vi "XML getApiRequest.vi"(11 "Formatted XML":string) -> (3 "PIM API Request":T1={"#attributes"={"xmlns"="http://www.summitekinstruments.com", "xmlns:xsi"="http://www.w3.org/2001/XMLSchema-instance", "xsi:schemaLocation"="http://www.summitekinstruments.com PIMXMLSchema.xsd"}, "Commands"={"#attributes"={"Token"="", "Legacy"=FALSE}, "Command"=[]}})   [LabVIEW 2011]
uses:
  Controls/PIM.API.REQUEST.ctl
  Controls/PIM.API.Command.Collection.ctl
  Controls/PIM.API.Command.Unique.ctl
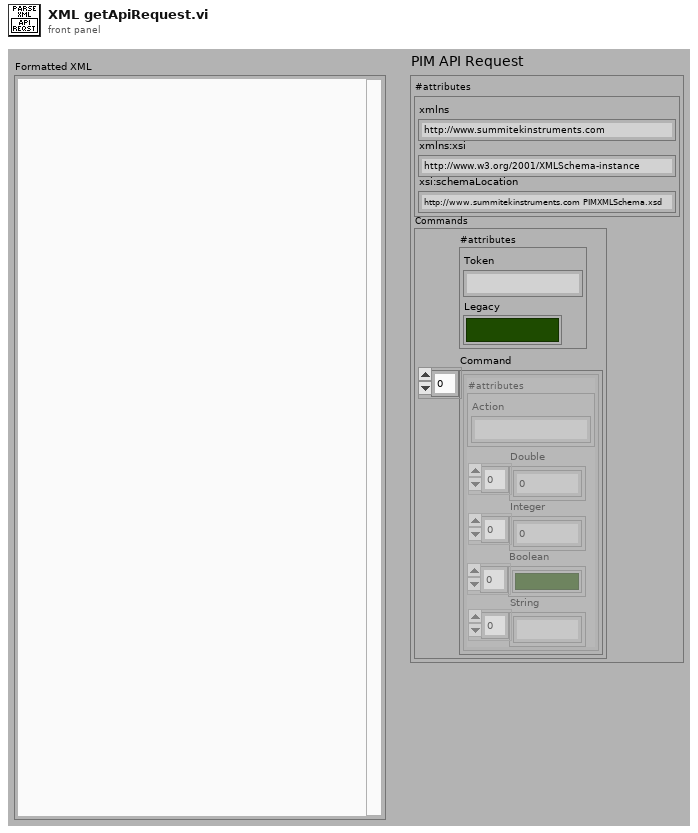
[diagram p1: front panel]
types:
  T1 = typedef "PIM.API.REQUEST.ctl" = cluster{"#attributes":cluster{"xmlns":string, "xmlns:xsi":string, "xsi:schemaLocation":string}, "Commands":T2}
  T2 = typedef "PIM.API.Command.Collection.ctl" = cluster{"#attributes":cluster{"Token":string, "Legacy":bool}, "Command":T3[]}
  T3 = typedef "PIM.API.Command.Unique.ctl" = cluster{"#attributes":cluster{"Action":string}, "Double":dbl[], "Integer":i32[], "Boolean":bool[], "String":string[]}
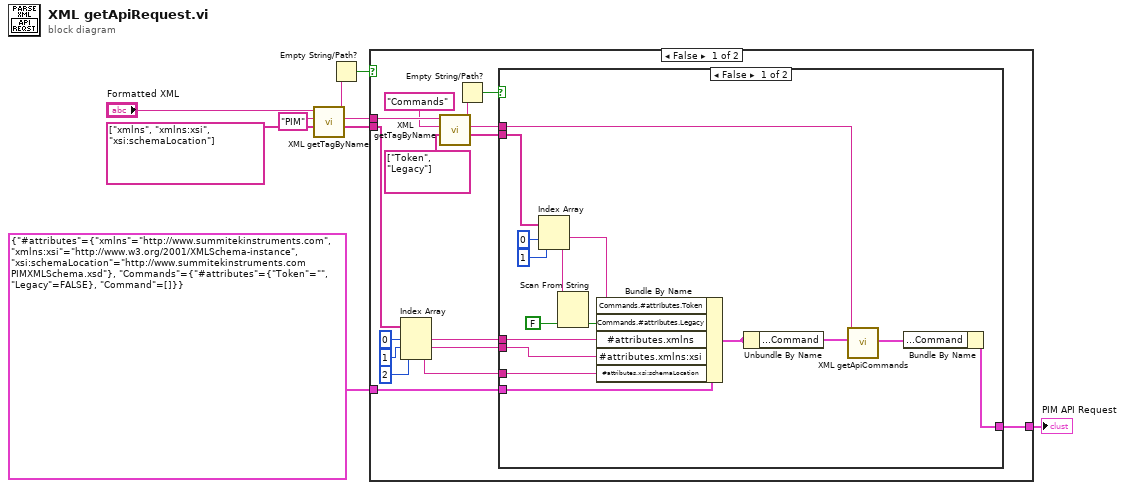
[diagram p0: block diagram]
diagram:
  n1 = call "XML getTagByName.vi"("Get Attributes"=string[] ["xmlns", "xmlns:xsi", "xsi:schemaLocation"], "Tag Name"="PIM", "XML String"="Formatted XML") -> ("Attribute Values"=w3:string[], "Tag Contents"=w2:string, "Matching Tag"=w1:string)  [unwired: 4 in, 2 out]
  n2 = Empty String/Path?(string/path=w1) -> (empty?=w9:bool)
  n3 = case shown="False" w9 {
    tunnel: T1 {"#attributes"={"xmlns"="http://www.summitekinstruments.com", "xmlns:xsi"="http://www.w3.org/2001/XMLSchema-instance", "xsi:schemaLocation"="http://www.summitekinstruments.com PIMXMLSchema.xsd"}, "Commands"={"#attributes"={"Token"="", "Legacy"=FALSE}, "Command"=[]}} ("PIM API Request") -> [w17 w43]
    tunnel: [w10 w43] -> w7
    tunnel: w2 -> [w25 _]
    tunnel: w3 -> [w21 _]
    frame False {
      n4 = Index Array(array=w21, index #1=0 ("index"), index #2=1 ("index"), index #3=2 ("index")) -> (element #1=w20:string, element #2=w19:string, element #3=w18:string)
      n5 = call "XML getTagByName.vi"("Get Attributes"=string[] ["Token", "Legacy"], "Tag Name"="Commands", "XML String"=w25) -> ("Attribute Values"=w13:string[], "Tag Contents"=w23:string, "Matching Tag"=w12:string)  [unwired: 4 in, 2 out]
      n6 = Empty String/Path?(string/path=w12) -> (empty?=w11:bool)
      n7 = case shown="False" w11 {
        tunnel: w23 -> [w26 _]
        tunnel: w20 -> [w41 _]
        tunnel: w19 -> [w40 _]
        tunnel: w18 -> [w39 _]
        tunnel: w17 -> [w38 w42]
        tunnel: w13 -> [w30 _]
        tunnel: [w27 w42] -> w10
        frame False {
          n8 = Index Array(array=w30, index #1=0 ("index"), index #2=1 ("index")) -> (element #1=w36:string, element #2=w33:string)
          n9 = Scan From String(input string=w33, default 1=FALSE ("Legacy")) -> (output 1=w32:bool)  [unwired: 3 in, 3 out]
          n10 = Bundle By Name(cluster=w38, "Commands.#attributes.Token"=w36, "Commands.#attributes.Legacy"=w32, "#attributes.xmlns"=w41, "#attributes.xmlns:xsi"=w40, "#attributes.xsi:schemaLocation"=w39) -> (w29:T1)
          n11 = Unbundle By Name(w29) -> ("Commands.Command"=w31:T3[])
          n12 = call "XML getApiCommands.vi"("Commands In"=w31, "Commands XML"=w26) -> ("Commands Out"=w28:T3[])  [unwired: 9 in]
          n13 = Bundle By Name(cluster=w29, "Commands.Command"=w28) -> (w27:T1)
        }
        frame True {
        }
      }
    }
    frame True {
      # "Tag Not Found"
    }
  }
  "PIM API Request" <- w7
